vi "SPI Write Read N Frames.vi"(5 "CS Configuration":T1, 7 "SPI Channel (0)":u8, 8 "Error In":errorcluster, 9 "SPI Frame Size":u8, 10 "Data":u8[](array[numeric]), 11 "LINX Resource":T3) -> (0 "Error Out":errorcluster, 2 "Read Data":u8[](array[numeric]), 3 "LINX Resource":T3, 4 "status":i32)   [LabVIEW 2020, in "LMH-LINX.lvlib"]
doc: "Transmit data on the specified SPI channel and read the response. This VI breaks the transmission up into multiple frames where each frame consists of setting CS active, shifting out a subset of the data bytes, then setting CS idle.\n\nSPI is full duplex, therefore the write and read operations take place simultaneously.\n\n<b>SPI Channel</b> specifies the SPI channel to write/read to.\n\n<b>Data</b> is a U8 array of data bytes to shift out starting with Data[0] to Data[n-1].\n\n<b>SPI Frame Size</b> specifies the number of bytes shifted out between toggling CS.\n\n<b>CS Channel</b> specifies the Chip Select (DIO) channel to use during the SPI transaction.\n\n<b>CS Logic Level</b> specifies the polarity of the chip select output. Active low is most common and results in CS starting in the idle/high state and data being trasnmitted after CS is driven to the active/low state."
uses:
  LMH-LINX.lvlib
  Private/Type Defs/LINX Ref.ctl
  Private/Type Defs/Platform.ctl
  Private/Type Defs/Interface.ctl
  Private/Device/Type Defs/LINX Device Config.ctl
  Private/Device/Type Defs/TCP Config.ctl
  Private/Device/Type Defs/Channels.ctl
  SPI CS Config.ctl
  Private/Type Defs/Peripherals/SPI/SPI CS Logic Level.ctl
  Private/Type Defs/Peripheral.ctl
  Private/Utilties/Generate Error.vi
  Private/Device/Device.lvlib
  Private/Local IO/Local IO.lvlib
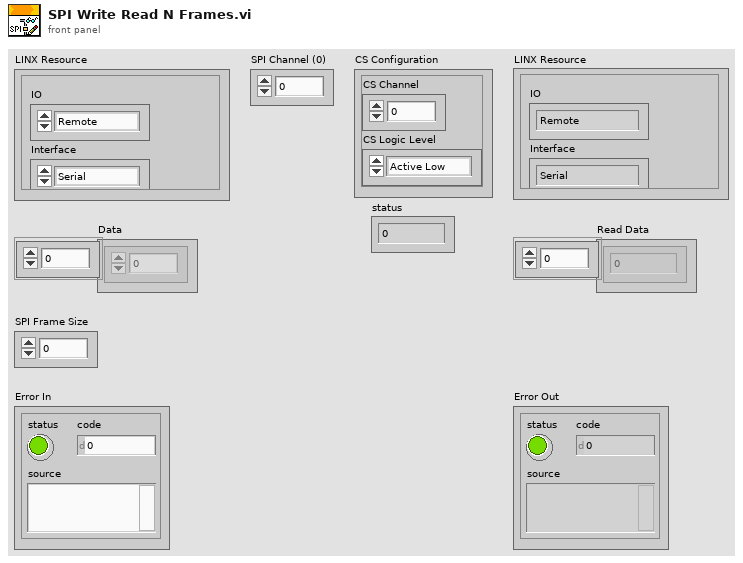
[diagram p1: front panel]
types:
  T1 = typedef "LMH-LINX.lvlib/SPI CS Config.ctl" = cluster{"CS Channel":u8, "CS Logic Level":T2}
  T2 = typedef "LMH-LINX.lvlib/SPI CS Logic Level.ctl" = enum8{"Active Low", "Active High"}
  T3 = typedef "LMH-LINX.lvlib/LINX Ref.ctl" = cluster{"IO":T4, "Interface":T5, "LINX Device Config":T6}
  T4 = typedef "LMH-LINX.lvlib/Platform.ctl" = enum16{"Remote", "Local"}
  T5 = typedef "LMH-LINX.lvlib/Interface.ctl" = enum16{"Serial", "TCP"}
  T6 = typedef "LMH-LINX.lvlib/Device.lvlib/LINX Device Config.ctl" = cluster{"Interface":T5, "COM Port":refnum<visa-resource-name>, "TCP Configuration":T7, "Device Family":u8, "Device ID":u8, "Device Name":string, "TCP Ref":refnum<k5>, "Channels":T8}
  T7 = typedef "LMH-LINX.lvlib/Device.lvlib/TCP Config.ctl" = cluster{"IP Address":string, "Port":u16}
  T8 = typedef "LMH-LINX.lvlib/Channels.ctl" = cluster{"DI":u8[], "DO":u8[], "AI":u8[], "AO":u8[], "PWM":u8[], "QE":u8[], "UART":u8[], "I2C 2":u8[], "SPI":u8[], "CAN":u8[], "Servo":u8[], "AI Ref (V)":dbl, "AI Resolution (Bits)":u8, "AO Ref (V)":dbl, "AO Resolution (Bits)":u8}
  T9 = typedef "LMH-LINX.lvlib/Peripheral.ctl" = enum8{"DI", "DO", "AI", "AO", "PWM", "QE", "UART", "I2C", "SPI", "CAN", "Servo"}
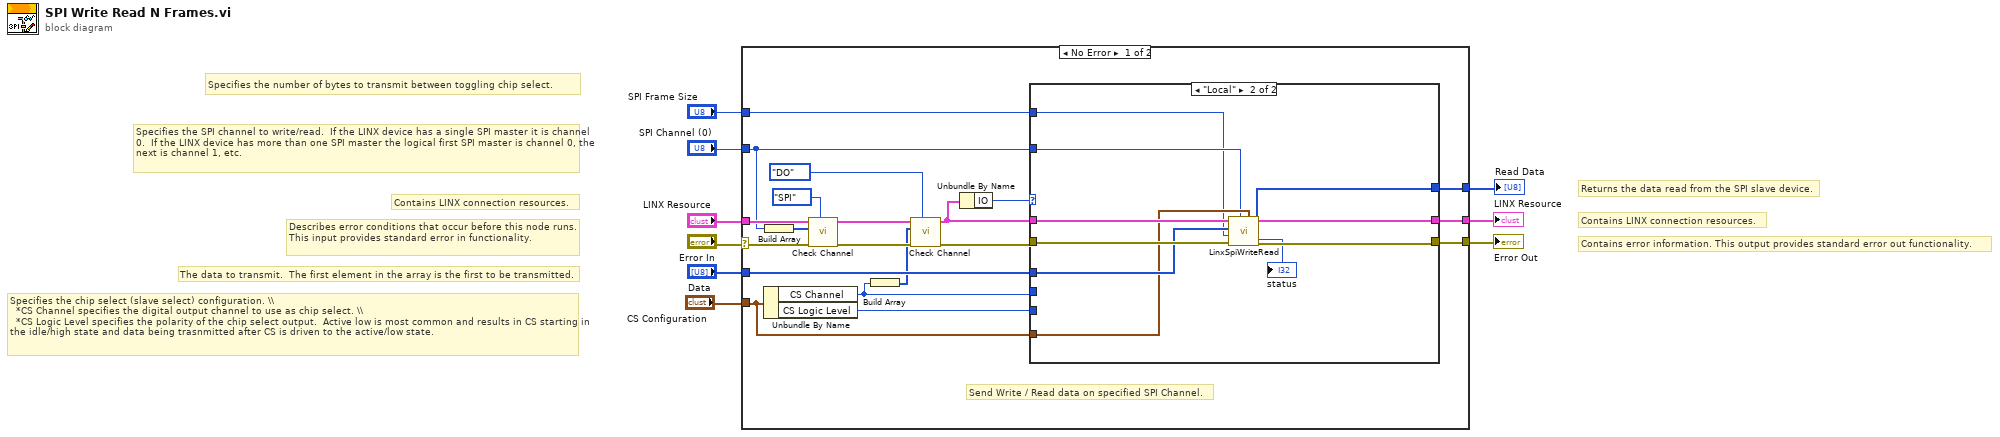
[diagram p0: block diagram]
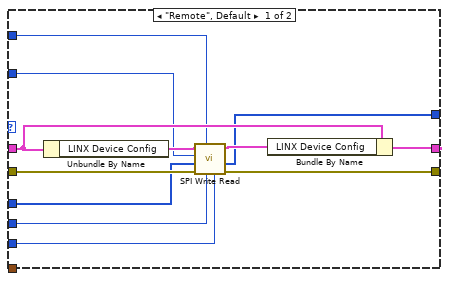
[diagram p2: hidden frame]
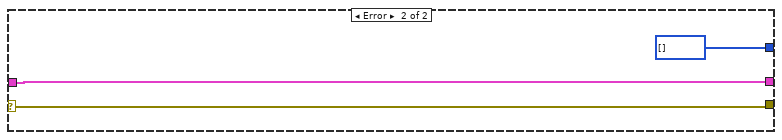
[diagram p3: hidden frame]
diagram:
  # "Returns the data read from the SPI slave device."
  # "Contains error information. This output provides standard error out functionality."
  # "Specifies the chip select (slave select) configuration. \\\\\n  *CS Channel specifies the digital output channel to use as chip select. \\\\ \n  *CS Logic Level specifies the polarity of the chip select output.  Active low is most common and results in CS starting in the idle/high state and data being trasnmitted after CS is driven to the active/low state."
  # "Specifies the number of bytes to transmit between toggling chip select."
  # "The data to transmit.  The first element in the array is the first to be transmitted."
  # "Specifies the SPI channel to write/read.  If the LINX device has a single SPI master it is channel 0.  If the LINX device has more than one SPI master the logical first SPI master is channel 0, the next is channel 1, etc."
  # "Contains LINX connection resources."
  # "Contains LINX connection resources."
  # "Describes error conditions that occur before this node runs. This input provides standard error in functionality."
  n1 = case shown="No Error" "Error In" {
    selector: "Error In" -> [w18 w54]
    tunnel: [w28 w54] -> w9
    tunnel: "LINX Resource" -> [w27 w52]
    tunnel: "SPI Channel (0)" -> [w25 _]
    tunnel: [w23 u8[] [] ("Frames Read")] -> w6
    tunnel: "Data" -> [w22 _]
    tunnel: "SPI Frame Size" -> [w21 _]
    tunnel: [w20 w52] -> w3
    tunnel: "CS Configuration" -> [w10 _]
    frame No Error {
      # "Send Write / Read data on specified SPI Channel."
      n2 = Unbundle By Name(w10) -> ("CS Channel"=w13:u8, "CS Logic Level"=w19:T2)
      n3 = Build Array(w25) -> (w26:u8[])
      n4 = call "Check Channel.vi"("Peripheral"=Peripheral."SPI", "Error In"=w18, "Channels"=w26, "LINX Resource"=w27) -> ("Error Out"=w17:errorcluster, "LINX Resource"=w15:T3)  [unwired: 5 in, 1 out]
      n5 = Build Array(w13) -> (w12:u8[])
      n6 = call "Check Channel.vi"("Peripheral"=Peripheral."DO", "Error In"=w17, "Channels"=w12, "LINX Resource"=w15) -> ("Error Out"=w16:errorcluster, "LINX Resource"=w14:T3)  [unwired: 5 in, 1 out]
      n7 = Unbundle By Name(w14) -> ("IO"=w29:T4)
      n8 = case shown="\"Local\"" w29 {
        tunnel: w16 -> [w39 w50]
        tunnel: w14 -> [w41 w51]
        tunnel: [w40 w44] -> w28
        tunnel: [w30 w45] -> w20
        tunnel: w25 -> [w34 w47]
        tunnel: [w36 w43] -> w23
        tunnel: w22 -> [w35 w49]
        tunnel: w21 -> [w33 w46]
        tunnel: w13 -> [w32 _]
        tunnel: w19 -> [w31 _]
        tunnel: w10 -> [_ w48]
        frame "Remote", Default {
          n9 = Unbundle By Name(w41) -> ("LINX Device Config"=w37:T6)
          n10 = call "SPI Write Read.vi"("CS Logic Level"=w31, "CS Pin (10)"=w32, "SPI Frame Size (1)"=w33, "Error In"=w39, "Data"=w35, "SPI Channel"=w34, "LINX Device Config"=w37) -> ("Error Out"=w40:errorcluster, "Read Data"=w36:u8[], "LINX Device Config"=w38:T6)  [unwired: 2 in]
          n11 = Bundle By Name(cluster=w41, "LINX Device Config"=w38) -> (w30:T3)
        }
        frame "Local" {
          n12 = call "LinxSpiWriteRead.vi"("CS Configuration"=w48, "SPI Channel"=w47, "Error In"=w50, "SPI Frame Size (0)"=w46, "Data"=w49, "LINX Resource"=w51) -> ("Error Out"=w44:errorcluster, "Data"=w43:u8[], "LINX Resource"=w45:T3, "status"=→"status":i32)  [unwired: 2 in]
        }
      }
    }
    frame Error {
    }
  }
  "Error Out" <- w9
  "LINX Resource" <- w3
  "Read Data" <- w6
